vi "state_response.vi"   [LabVIEW 2020]
uses:
  New folder/Control 1.ctl
types:
  T1 = typedef "Control 1.ctl" = enum16{"GF Home", "Home Back", "Long Drive", "Dinner", "Home M", "Temple", "Office", "Meeting", "GF", "Club", "Movie"}
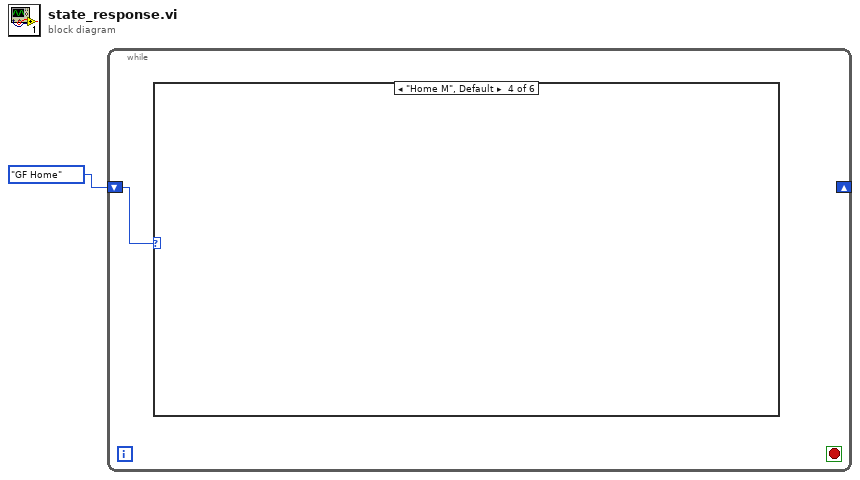
[diagram p0: block diagram]
diagram:
  n1 = while {
    shift-right: _ -> [_]
    shift-left: Control_1."GF Home" -> [w2]
    stop <- _ stop-if-true
    n2 = case shown="\"Home M\", Default" w2 {
      frame "GF Home" {
      }
      frame "Long Drive" {
      }
      frame "Dinner" {
      }
      frame "Home M", Default {
      }
      frame "Temple" {
      }
      frame "Home Back" {
      }
    }
  }
